vi "StateSpaceUtil_MakeCovarianceMatrix.vi"(7 "States":i32, 11 "StdDevs":T1) -> (0 "Size Coerced":bool, 3 "Covariance Matrix":T1)   [LabVIEW 2019, in "Trajectory_Library.lvlib"]
doc: "Creates a new LINEAR SYSTEM data cluster with the specified values. \n\n\nInputs: \n - XXX -- XXX.\n\nOutputs:\n - XXX -- XXX."
uses:
  Trajectory_Library.lvlib
  <vilib>/Analysis/Matrix/Datatypes/RealMatrix.ctl
  <vilib>/Analysis/Matrix/NI_Matrix.lvlib
panel:
  # "<States,States>"
  # "<States,1>"
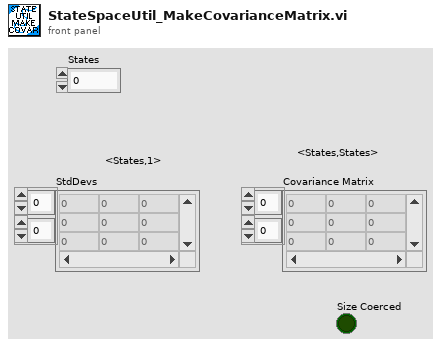
[diagram p1: front panel]
types:
  T1 = typedef "NI_Matrix.lvlib/RealMatrix.ctl" = dbl[][]
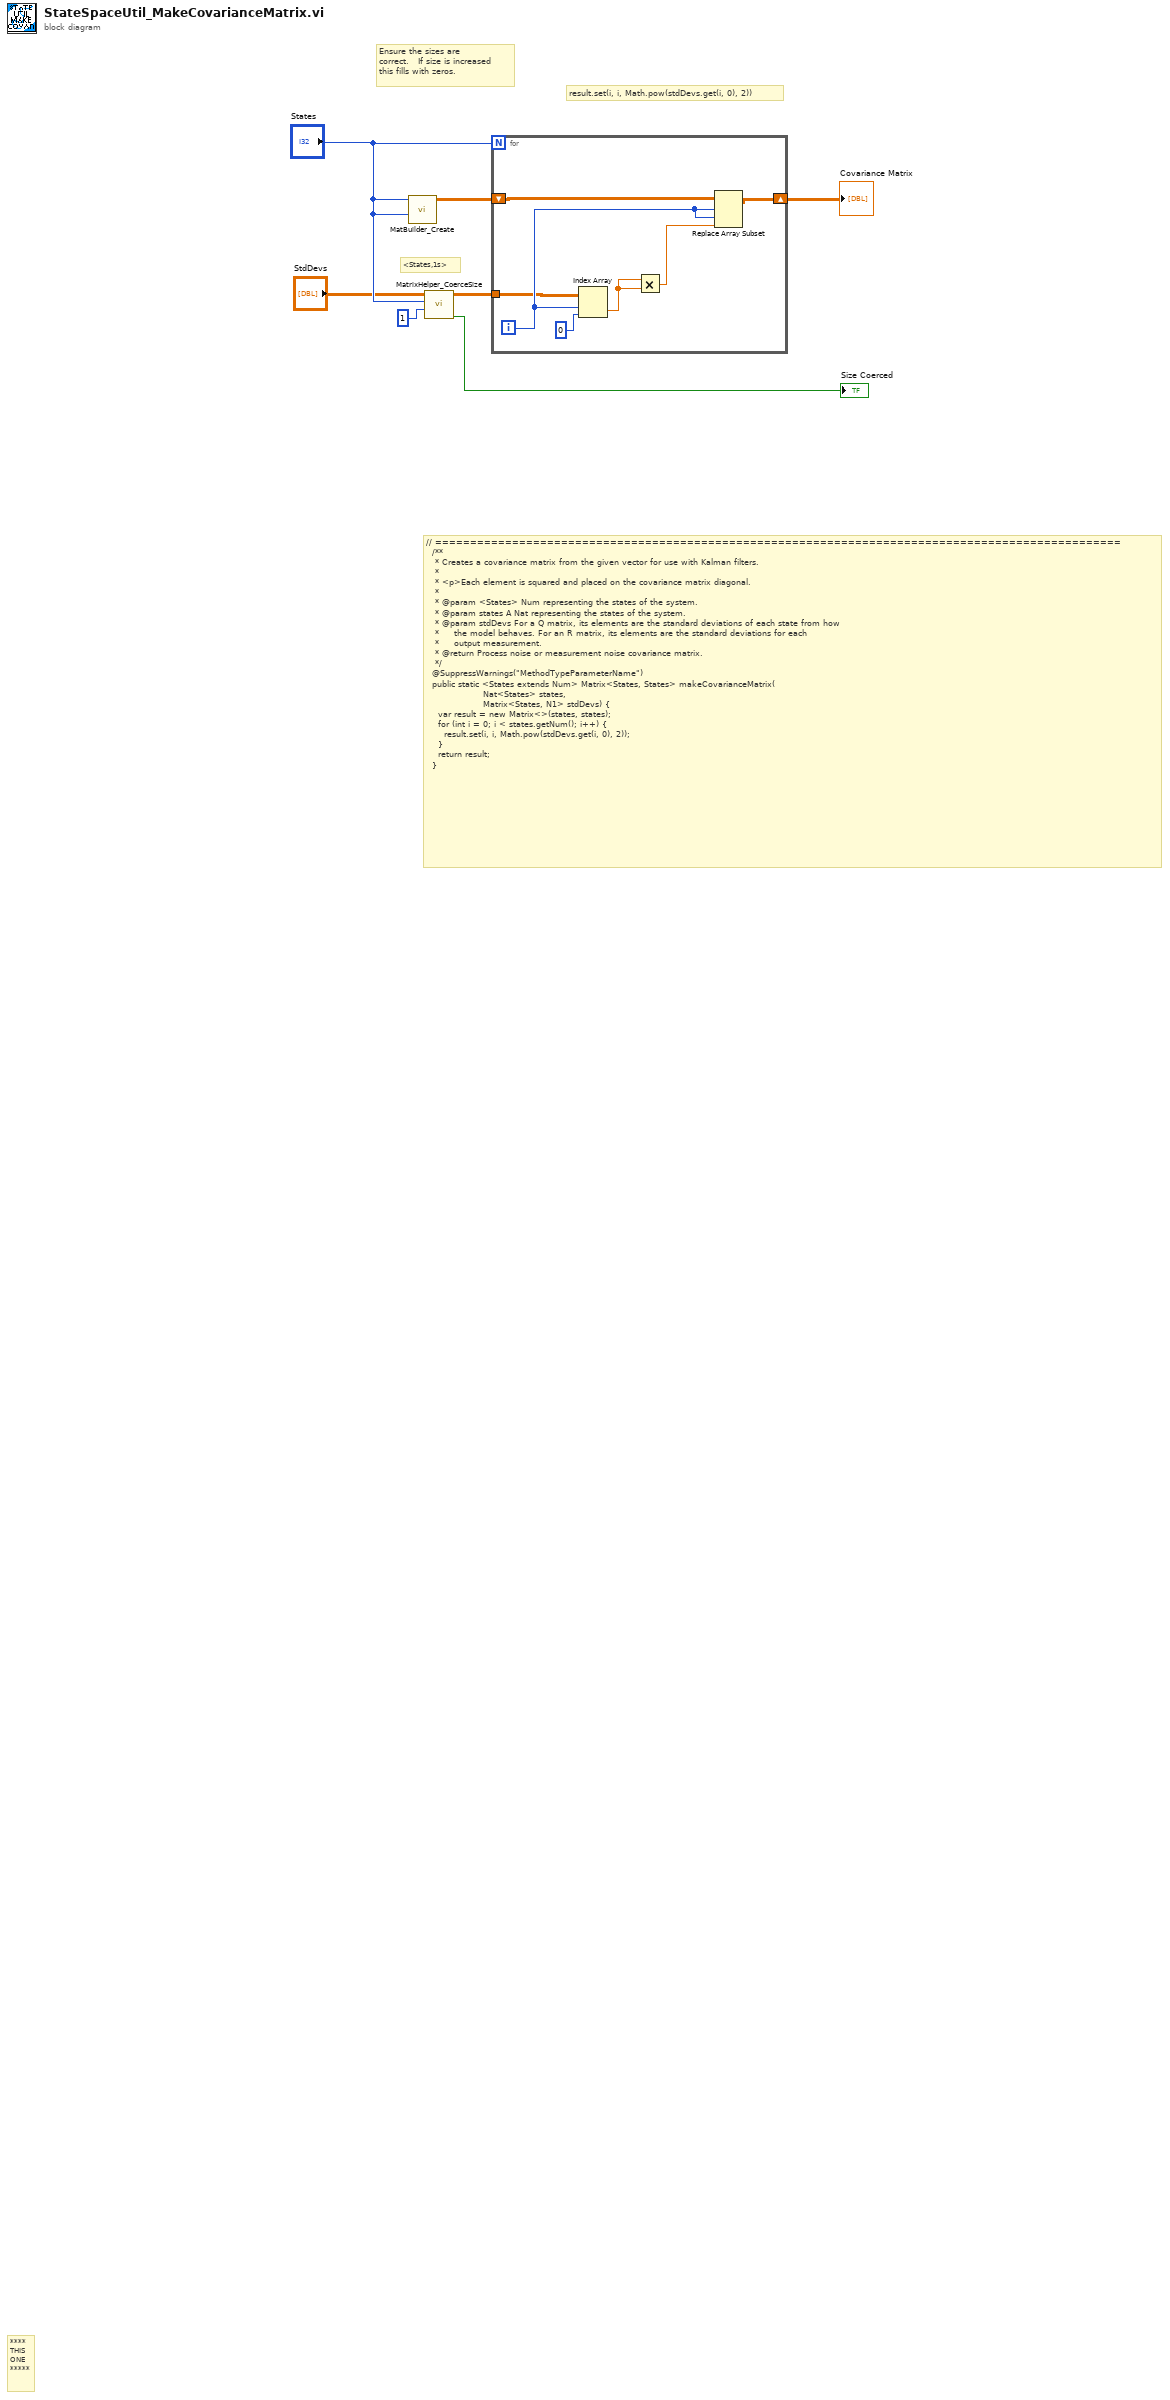
[diagram p0: block diagram]
diagram:
  # "// ==================================================================================================\n  /**\n   * Creates a covariance matrix from the given vector for use with Kalman filters.\n   *\n   * <p>Each element is squared and placed on the covariance matrix diagonal.\n   *\n   * @param <States> Num representing the states of the system.\n   * @param states A Nat representing the states of the system.\n   * @param stdDevs For a Q matrix, its elements are the standard deviations of each state from how\n   *     the model behaves. For an R matrix, its elements are the standard deviations for each\n   *     output measurement.\n   * @return Process noise or measurement noise covariance matrix.\n   */\n  @SuppressWarnings(\"MethodTypeParameterName\")\n  public static <States extends Num> Matrix<States, States> makeCovarianceMatrix(\n                   Nat<States> states, \n                   Matrix<States, N1> stdDevs) {\n    var result = new Matrix<>(states, states);\n    for (int i = 0; i < states.getNum(); i++) {\n      result.set(i, i, Math.pow(stdDevs.get(i, 0), 2));\n    }\n    return result;\n  }"
  # "result.set(i, i, Math.pow(stdDevs.get(i, 0), 2))"
  # "<States,1s>"
  # "Ensure the sizes are\ncorrect.   If size is increased \nthis fills with zeros."
  # "****\nTHIS\nONE\n*****"
  n1 = call "MatBuilder_Create.vi"("Columns"="States", "Rows"="States") -> ("output matrix"=w6:T1)  [unwired: 9 in]
  n2 = call "MatrixHelper_CoerceSize.vi"("Columns"=1 ("number of columns"), "Rows"="States", "input matrix"="StdDevs") -> ("Coerced"=→"Size Coerced":bool, "output matrix"=w3:T1)  [unwired: 7 in]
  n3 = for {
    N: "States" -> [_]
    tunnel: w3 -> [w10]
    shift-right: [w14] -> w7
    shift-left: w6 -> [w13]
    i -> [w12]
    n4 = Index Array(array=w10, index (row)=w12, index (col)=0) -> (element=w9:dbl)
    n5 = Multiply(x=w9, y=w9) -> (x*y=w8:dbl)
    n6 = Replace Array Subset(array=w13, new element=w8, index (row)=w12, index (col)=w12) -> (w14:T1)
  }
  "Covariance Matrix" <- w7
